vi "Winch State Transition Example.vi"() -> ()   [LabVIEW 2016]
uses:
  Global State Variables.vi
panel:
  out "WinchState":enum16{"WinchOff", "WinchClimb", "WinchHold"}(ring)
  in  "Button Ignore Timer":dbl
  in  "stop":bool
  in  "State Selector Methods":enum32{"using one button", "using two buttons"}(tab)
  in  "single buton selector":bool
  in  "right button\nselector":bool
  in  "left button \nselector":bool
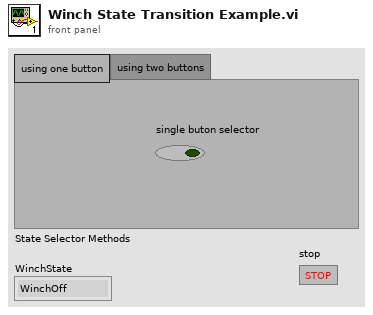
[diagram p1: front panel]
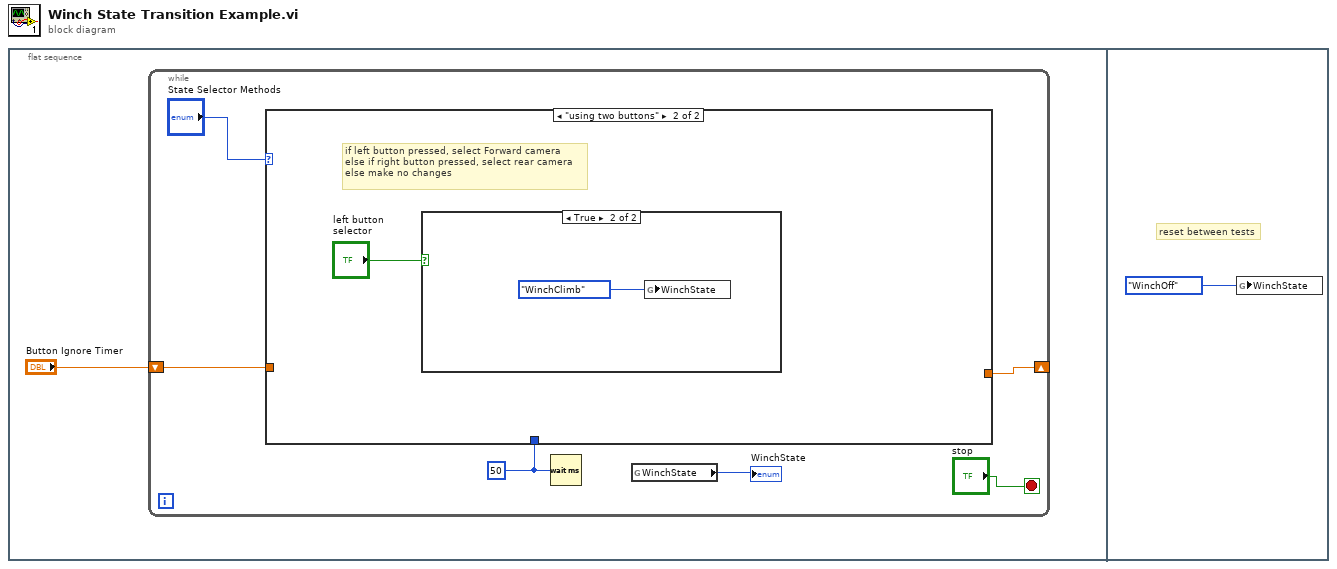
[diagram p0: block diagram]
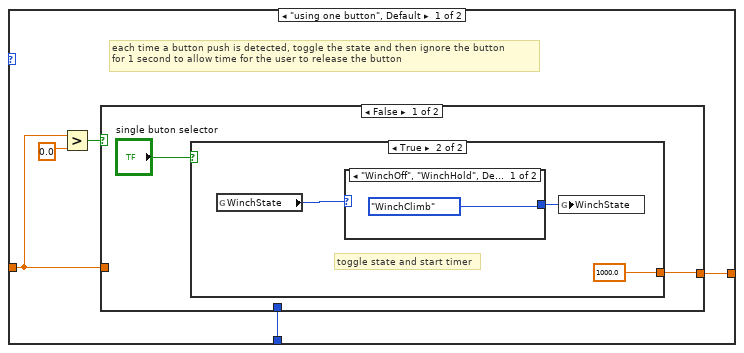
[diagram p2: hidden frame]
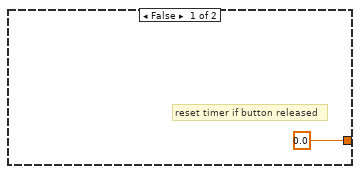
[diagram p3: hidden frame]
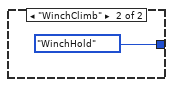
[diagram p4: hidden frame]
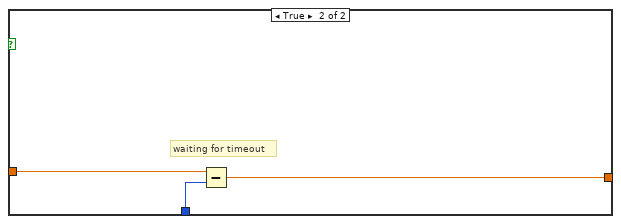
[diagram p5: hidden frame]
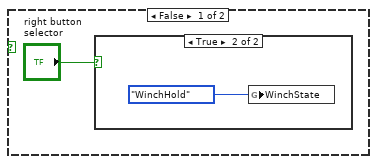
[diagram p6: hidden frame]
diagram:
  n1 = flat-sequence {
    frame #0 {
      n2 = while {
        shift-right: [w3] -> _
        shift-left: "Button Ignore Timer" -> [w5]
        stop <- "stop" stop-if-true
        w4 = u32 50 ("milliseconds to wait")
        n3 = case shown="\"using two buttons\"" "State Selector Methods" {
          tunnel: w5 -> [w10 _]
          tunnel: w4 -> [w9 _]
          tunnel: [w8 _] -> w3
          frame "using one button", Default {
            # "each time a button push is detected, toggle the state and then ignore the button \nfor 1 second to allow time for the user to release the button"
            n4 = Greater?(x=w10, y=0.0) -> (0:w12:bool)
            n5 = case shown="False" w12 {
              tunnel: w10 -> [_ w22]
              tunnel: w9 -> [_ w23]
              tunnel: [w13 w21] -> w8
              frame False {
                n6 = case shown="True" "single buton selector" {
                  tunnel: [0.0 ("Button Ignore Timer") 1000.0] -> w13
                  frame False {
                    # "reset timer if button released"
                  }
                  frame True {
                    # "toggle state and start timer"
                    n7 = global read "Global State Variables.vi" "WinchState"() -> (w18:enum16{"WinchOff", "WinchClimb", "WinchHold"})
                    n8 = case shown="\"WinchOff\", \"WinchHold\", Default" w18 {
                      tunnel: [enum16{"WinchOff", "WinchClimb", "WinchHold"}."WinchClimb" ("WinchState") enum16{"WinchOff", "WinchClimb", "WinchHold"}."WinchHold" ("WinchState")] -> w16
                      frame "WinchOff", "WinchHold", Default {
                      }
                      frame "WinchClimb" {
                      }
                    }
                    n9 = global write "Global State Variables.vi" "WinchState"(w16) -> ()
                  }
                }
              }
              frame True {
                # "waiting for timeout"
                n10 = Subtract(x=w22, y=w23) -> (x-y=w21:dbl)
              }
            }
          }
          frame "using two buttons" {
            # "if left button pressed, select Forward camera\nelse if right button pressed, select rear camera\nelse make no changes"
            n11 = case shown="True" "left button \nselector" {
              frame False {
                n12 = case shown="True" "right button\nselector" {
                  frame False {
                  }
                  frame True {
                    n13 = global write "Global State Variables.vi" "WinchState"(enum16{"WinchOff", "WinchClimb", "WinchHold"}."WinchHold" ("WinchState")) -> ()
                  }
                }
              }
              frame True {
                n14 = global write "Global State Variables.vi" "WinchState"(enum16{"WinchOff", "WinchClimb", "WinchHold"}."WinchClimb" ("WinchState")) -> ()
              }
            }
          }
        }
        n15 = Wait (ms)(milliseconds to wait=w4) -> ()  [unwired: 1 out]
        n16 = global read "Global State Variables.vi" "WinchState"() -> (→"WinchState":enum16{"WinchOff", "WinchClimb", "WinchHold"})
      }
    }
    frame #1 {
      # "reset between tests"
      n17 = global write "Global State Variables.vi" "WinchState"(enum16{"WinchOff", "WinchClimb", "WinchHold"}."WinchOff" ("WinchState")) -> ()
    }
  }
